vi "Read Payload.vi"(8 "error in (no error)":errorcluster, 9 "Timeout ms (0)":i32, 11 "Basic WebSocket Manager in":refnum<class "Basic WebSocket Manager.lvclass">) -> (0 "error out":errorcluster, 1 "Timeout":bool, 2 "WS Payload":T1, 3 "Basic WebSocket Manager out":refnum<class "Basic WebSocket Manager.lvclass">)   [LabVIEW 2020, in "HTTP Server.lvlib" / "Basic WebSocket Manager.lvclass"]
uses:
  Basic WebSocket Manager.lvclass
  Basic WebSocket Manager.lvclass/Basic WebSocket Manager.ctl
  WebSocket Format.ctl
  HTTP Server.lvlib
  WS Payload.ctl
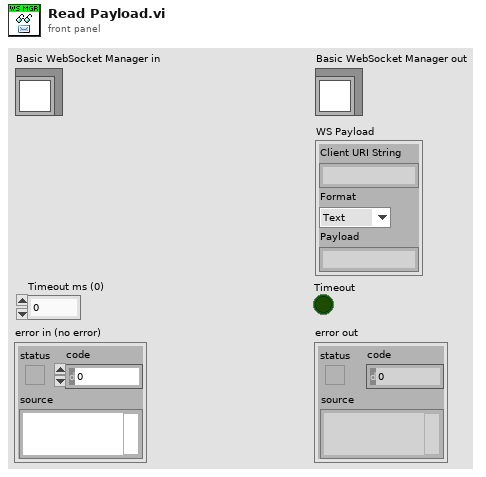
[diagram p1: front panel]
types:
  T1 = typedef "HTTP Server.lvlib/Basic WebSocket Manager.lvclass/WS Payload.ctl" = cluster{"Client URI String":string, "Format":T2, "Payload":string}
  T2 = typedef "HTTP Server.lvlib/WebSocket Format.ctl" = enum16{"Text", "Binary"}
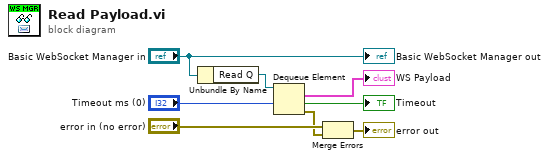
[diagram p0: block diagram]
diagram:
  n1 = Unbundle By Name("Basic WebSocket Manager in") -> ("Read Q"=w6:refnum<queue>)
  n2 = Dequeue Element(queue=w6, timeout in ms (-1)="Timeout ms (0)") -> (element=→"WS Payload":T1, timed out?=→"Timeout":bool, error out=w1:errorcluster)  [unwired: 1 in, 1 out]
  n3 = Merge Errors("error in (no error)", w1) -> (→"error out":errorcluster)
  "Basic WebSocket Manager out" <- "Basic WebSocket Manager in"
